vi "Initialize.vi"(8 "error in (no error)":errorcluster, 10 "Array of Hardware":refnum<class "Hardware.lvclass">[](array[class]), 11 "VacuumLine in":refnum<class "VacuumLine.lvclass">) -> (0 "error out":errorcluster, 2 "duplicate LogicIO labels?":bool, 3 "VacuumLine out":refnum<class "VacuumLine.lvclass">)   [LabVIEW 2016, in "Hardware.lvlib" / "VacuumLine.lvlib" / "VacuumLine.lvclass"]
uses:
  <userlib>/Common Components/Hardware/Abstract System/VacuumLine/VacuumLine/VacuumLine.lvclass
  <userlib>/Common Components/Hardware/Abstract Hardware/Hardware.lvclass
  <userlib>/Common Components/Hardware/Motor/Motor/Motor.lvclass
  <userlib>/Common Components/Hardware/Displacement Sensor/DispSnsr/DispSnsr.lvclass
  <userlib>/Common Components/Hardware/LogicIO/LogicIO/LogicIO.lvclass
  <userlib>/Common Components/Hardware/Abstract Hardware/Hardware.lvclass/Hardware.ctl
  <userlib>/Common Components/Hardware/Abstract System/VacuumLine/VacuumLine/VacuumLine.lvclass/VacuumLine.ctl
  <userlib>/Common Components/Hardware/Abstract Hardware/Read Label.vi
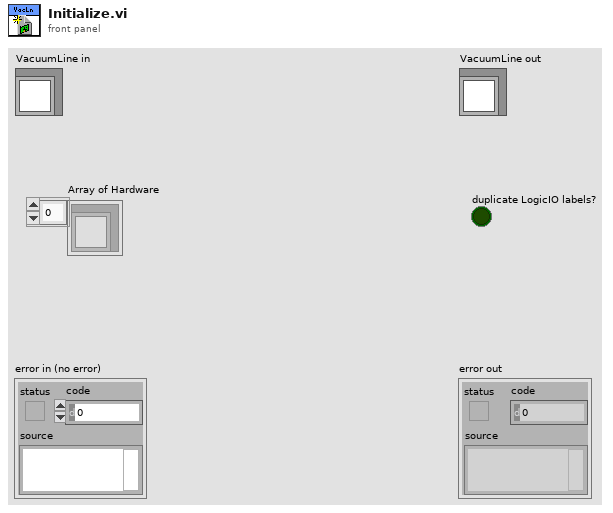
[diagram p1: front panel]
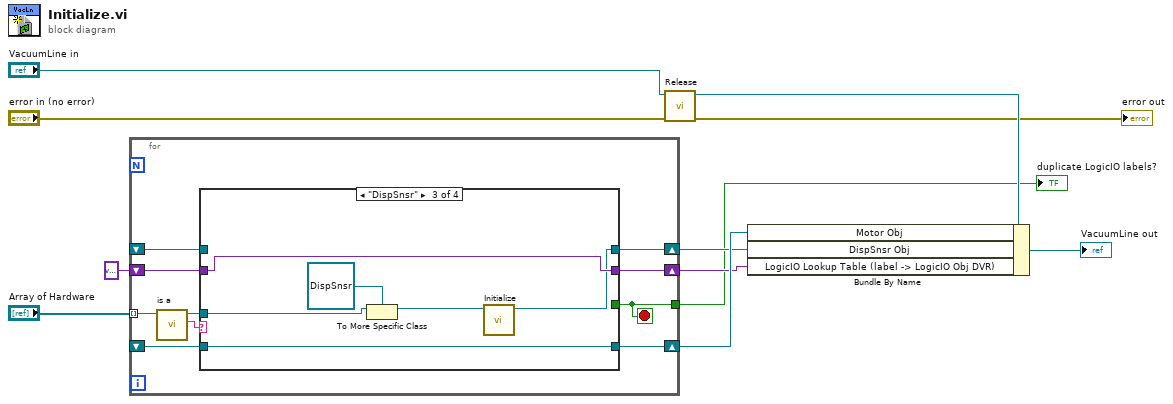
[diagram p0: block diagram]
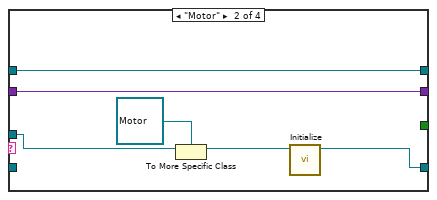
[diagram p3: hidden frame]
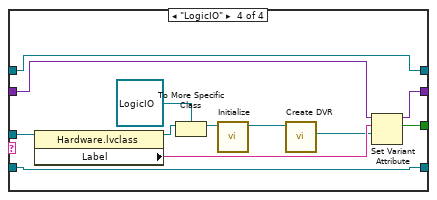
[diagram p4: hidden frame]
diagram:
  n1 = for {
    tunnel: "Array of Hardware" -> [w18] mode=indexing
    shift-right: [w20] -> w5
    shift-left: variant -> [w21]
    tunnel: [w19] -> w4
    shift-right: [w15] -> w7
    shift-left: _ -> [w14]
    shift-right: [w13] -> w6
    shift-left: _ -> [w12]
    stop <- w19 stop-if-true
    n2 = call-dynamic "is a.vi"("Hardware in"=w18) -> ("is a"=w16:string, "Hardware out"=w17:refnum<class "Hardware.lvclass">)  [unwired: 8 in, 1 out]
    n3 = case shown="\"DispSnsr\"" w16 {
      tunnel: w21 -> [w24 w30 w36 w48]
      tunnel: [w24 w30 w36 w47] -> w20
      tunnel: [_ _ _ w45] -> w19
      tunnel: w17 -> [_ w29 w34 w44]
      tunnel: [w23 w25 w35 w43] -> w15
      tunnel: w14 -> [w23 _ w35 w43]
      tunnel: [w22 w28 w31 w40] -> w13
      tunnel: w12 -> [w22 w28 _ w40]
      frame Default {
      }
      frame "Motor" {
        n4 = To More Specific Class(target class=refnum<class "Motor.lvclass"> refnum ("Hardware.lvlib:Motor.lvlib:Motor.lvclass"), reference=w29) -> (specific class reference=w26:refnum<class "Motor.lvclass">)  [unwired: 1 in, 1 out]
        n5 = call-dynamic "Initialize.vi"("CCD in"=w26) -> ("CCD out"=w25:refnum<class "Motor.lvclass">)  [unwired: 9 in, 1 out]
      }
      frame "DispSnsr" {
        n6 = To More Specific Class(target class=refnum<class "DispSnsr.lvclass"> refnum ("Hardware.lvlib:Displacement Sensor.lvlib:DispSnsr.lvclass"), reference=w34) -> (specific class reference=w32:refnum<class "DispSnsr.lvclass">)  [unwired: 1 in, 1 out]
        n7 = call-dynamic "Initialize.vi"("Hardware in"=w32) -> ("Hardware out"=w31:refnum<class "DispSnsr.lvclass">)  [unwired: 9 in, 1 out]
      }
      frame "LogicIO" {
        n8 = property class="Hardware.lvclass"(reference=w44) -> (reference out=w42:refnum<class "Hardware.lvclass">, "Label"=w46:string)  [unwired: 1 in, 1 out]
        n9 = To More Specific Class(target class=refnum<class "LogicIO.lvclass"> refnum ("Hardware.lvlib:LogicIO.lvlib:LogicIO.lvclass"), reference=w42) -> (specific class reference=w39:refnum<class "LogicIO.lvclass">)  [unwired: 1 in, 1 out]
        n10 = call-dynamic "Initialize.vi"("LogicIO in"=w39) -> ("LogicIO out"=w38:refnum<class "LogicIO.lvclass">)  [unwired: 9 in, 1 out]
        n11 = call <userlib>:"Create DVR.vi"("LogicIO in"=w38) -> ("data value reference"=w37:refnum<data-value>)  [unwired: 8 in, 2 out]
        n12 = Set Variant Attribute(Variant=w48, name=w46, value=w37) -> (Variant out=w47:variant, replaced=w45:bool)  [unwired: 1 in, 1 out]
      }
    }
  }
  "duplicate LogicIO labels?" <- w4
  n13 = call <userlib>:"Release.vi"("error in (no error)"="error in (no error)", "VacuumLine in"="VacuumLine in") -> ("error out"=→"error out":errorcluster, "VacuumLine out"=w10:refnum<class "VacuumLine.lvclass">)  [unwired: 8 in]
  n14 = Bundle By Name(cluster=w10, "Motor Obj"=w7, "DispSnsr Obj"=w6, "LogicIO Lookup Table (label -> LogicIO Obj DVR)"=w5) -> (→"VacuumLine out":refnum<class "VacuumLine.lvclass">)
